vi "Clear Driver VIs Dependent File Paths - 331.vi"(8 "error in (no error)":errorcluster, 11 "Device Item Ref in in":T1 format="%.0x") -> (0 "error out":errorcluster, 3 "Device Item Ref out":T1 format="%.0x")   [LabVIEW 2018, in "FPGA Addon Shared.lvlib"]
uses:
  FPGA Addon Shared.lvlib
  <vilib>/NI Veristand/Custom Device API/Custom Device Item Ref.ctl
  <vilib>/NI Veristand/Custom Device API/Custom Device API.lvlib
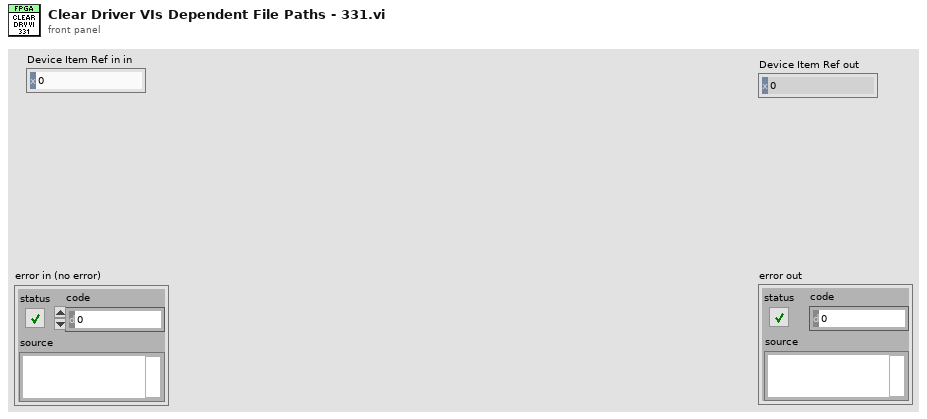
[diagram p1: front panel]
types:
  T1 = typedef "Custom Device API.lvlib/Custom Device Item Ref.ctl" = u64
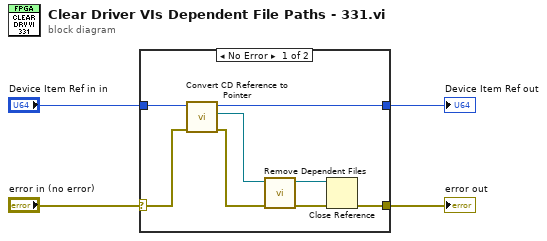
[diagram p0: block diagram]
diagram:
  n1 = case shown="No Error" "error in (no error)" {
    selector: "error in (no error)" -> [w10 w13]
    tunnel: [w5 w13] -> w3
    tunnel: "Device Item Ref in in" -> [w12 w14]
    tunnel: [w6 w14] -> w1
    frame No Error {
      n2 = call "Convert CD Reference to Pointer.vi"("error in (no error)"=w10, "Item Ref in"=w12) -> ("error out"=w9:errorcluster, ".NET Refnum out"=w11:refnum<k24>, "Item Ref out"=w6:T1)  [unwired: 7 in]
      n3 = call "Remove Dependent Files.vi"("error in (no error)"=w9, ".NET Refnum in"=w11) -> ("error out"=w7:errorcluster, ".NET Refnum out"=w8:refnum<k24>)  [unwired: 8 in]
      n4 = Close Reference(reference=w8, error in (no error)=w7) -> (error out=w5:errorcluster)
    }
    frame Error {
    }
  }
  "Device Item Ref out" <- w1
  "error out" <- w3
